vi "EncoderConfigurationSubVI.vi"(8 "error in":errorcluster, 10 "Input Terminal":tag, 11 "Counter physical channel":tag) -> (0 "error out":errorcluster, 3 "task out":refnum<k21>)   [LabVIEW 2017]
uses:
  <vilib>/DAQmx/create/channels.llb/DAQmx Create Channel (CI-Count Edges).vi
  <resource>/objmgr/daqmx.rc
panel:
  # "Task out"
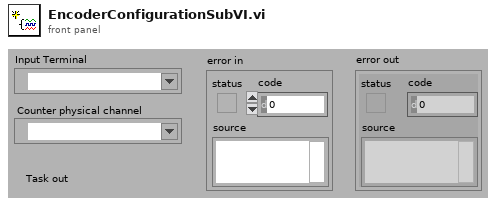
[diagram p1: front panel]
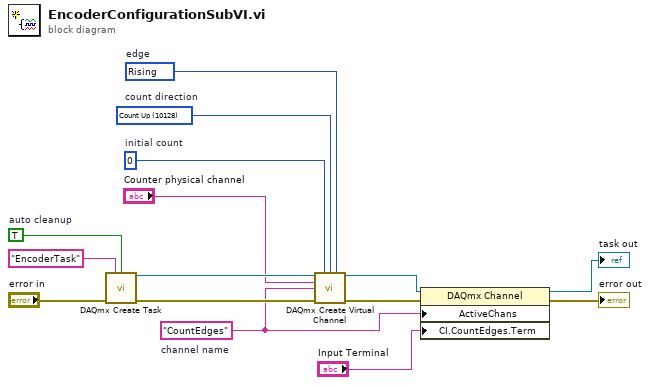
[diagram p0: block diagram]
diagram:
  w8 = 10280 items=["Rising"=10280, "Falling"=10171]  # edge
  w9 = 10128 items=["Count Up"=10128, "Count Down"=10124, "Externally Controlled"=10326]  # count direction
  w10 = u32 0  # initial count
  w4 = "CountEdges"  # channel name
  w13 = TRUE  # auto cleanup
  n1 = call <vilib>:"DAQmx Create Task.vi"("new task name"="EncoderTask", "auto cleanup"=w13, "error in"="error in") -> ("task out"=w12:refnum<k21>, "error out"=w14:errorcluster)  [unwired: 11 in]
  n2 = call-poly <vilib>:"DAQmx Create Virtual Channel.vi"("task in"=w12, "initial count"=w10, "count direction"=w9, "edge"=w8, "counter"="Counter physical channel", "name to assign"=w4, "error in"=w14) -> ("task out"=w6:refnum<k21>, "error out"=w11:errorcluster)  [unwired: 7 in]
  n3 = property class="DAQmx Channel"(reference=w6, error in=w11, "ActiveChans"=w4, "CI.CountEdges.Term"="Input Terminal") -> (reference out=→"task out":refnum<k21>, error out=→"error out":errorcluster)
